vi "Save Data Dialog.vi"() -> (1 "cancelled":bool, 2 "selected path":path)   [LabVIEW 2023]
uses:
  User_Vi/Settings.vi
panel:
  out "error out":errorcluster
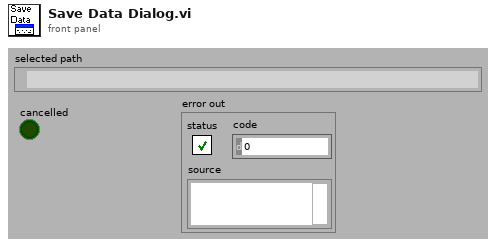
[diagram p1: front panel]
types:
  T1 = enum16{"Left Button", "Center Button", "Right Button", "Window Close"}
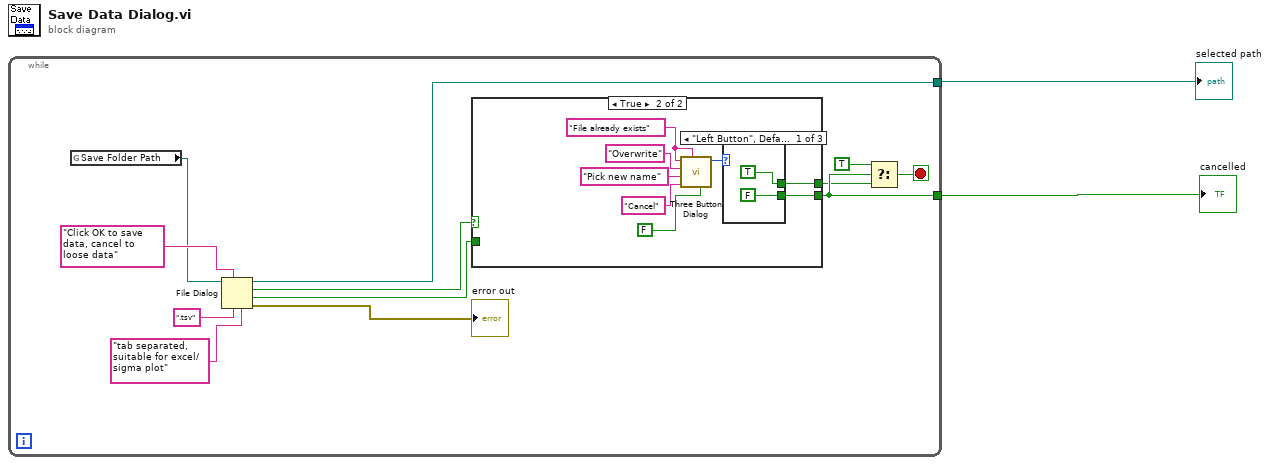
[diagram p0: block diagram]
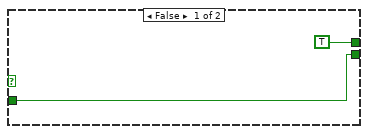
[diagram p2: hidden frame]
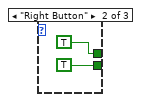
[diagram p3: hidden frame]
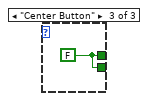
[diagram p4: hidden frame]
diagram:
  n1 = while {
    tunnel: [w8] -> w2
    tunnel: [w11] -> w1
    stop <- w7 stop-if-true
    n2 = global read "Settings.vi" "Save Folder Path"() -> (w3:path)
    n3 = File Dialog(4:"tab separated, suitable for excel/sigma plot", 6:".tsv", 7:"Click OK to save data, cancel to loose data", 11:w3) -> (0:→"error out":errorcluster, 1:w9:bool, 2:w10:bool, 3:w11:path)  [unwired: 1 in, 2 out]
    n4 = case shown="True" w10 {
      tunnel: w9 -> [w15 _]
      tunnel: [TRUE w18] -> w5
      tunnel: [w15 w17] -> w8
      frame False {
      }
      frame True {
        w23 = "File already exists" ("message")
        n5 = call <vilib>:"Three Button Dialog.vi"("Allow user to close window? (TRUE)"=FALSE, "Window Title (\"\")"=w23, "Right Button Text (\"Cancel\")"="Cancel" ("Right Button Text (\"Cancel\")"), "Center Button Text (\"No\")"="Pick new name" ("Center Button Text (\"No\")"), "Left Button Text (\"Yes\")"="Overwrite" ("T button name (\"OK\")"), "message"=w23) -> ("Which Button?"=w19:T1)  [unwired: 5 out]
        n6 = case shown="\"Left Button\", Default" w19 {
          tunnel: [TRUE ("Allow user to close window? (TRUE)") TRUE w29] -> w18
          tunnel: [FALSE TRUE w29] -> w17
          frame "Left Button", Default {
          }
          frame "Right Button" {
          }
          frame "Center Button" {
            w29 = FALSE
          }
        }
      }
    }
    n7 = Select(t=TRUE, s=w8, f=w5) -> (s? t:f=w7:bool)
  }
  "cancelled" <- w2
  "selected path" <- w1
